vi "NI-USB6509.vi"() -> ()   [LabVIEW 2020]
uses:
  <vilib>/Utility/miscctls.llb/LVPointTypeDef.ctl
  LabVIEW 2020 Toolkits/toolkits_lv2020_32bit/Synchronization.llb/SynchRefs_SetGet.ctl
  LabVIEW 2020 Toolkits/VI Server Toolkit/VI Server Libraries/VI Server_GetControl.llb/VI Server_STR_Get.vi
  LabVIEW 2020 Toolkits/VI Server Toolkit/VI Server Libraries/VI Server_Set Controls.llb/Set STR Control.vi
  LabVIEW 2020 Toolkits/VI Server Toolkit/VI Server Libraries/VI Server_GetControl.llb/VI Server_DAQmx_Device_Get.vi
  LabVIEW 2020 Toolkits/VI Server Toolkit/VI Server Toolkit LV2013.lvlib
panel:
  out "System.Message":string caption="System Message"
  in  "Help":bool
  in  "FP.Hide":bool caption="FrontPanel.Hide"
  in  "EXIT":bool
  in  "Tab.Main":enum32{"Digital I/O", "SETTINGS"}(tab)
  in  "DI.Port.Update":bool
  out "DI.Port.Lines.0:7":u8 caption="Port&Lines 7:0" format="%08b"
  in  "DI.Port":tag="Dev1/port0/line0:7" caption="Port"
  in  "DI.Line":tag="Dev1/port0/line0:7" caption="Line"
  in  "DI.Line.Update":bool caption="Update:"
  in  "DO.Port.Mask.Apply":bool
  in  "DO.Port.Lines.7:0.Mask":u8 caption="Port&Lines 7:0" format="%08b"
  out "DO.Port.State.Verify":bool caption="Verified"
  out "DO.Line.State.Verify":bool caption="Verified"
  in  "DO.Line.State":bool caption="State"
  in  "DO.Line":tag="Dev1/port0/line0:7" caption="Line"
  in  "DO.Port.Update":bool
  in  "DO.Port.Lines.7:0":u8 caption="Port&Lines 7:0" format="%08b"
  in  "DO.Port":tag="Dev1/port0/line0:7" caption="Port"
  in  "DO.Line.Update":bool caption="Update:"
  out "DI.Line.State":bool caption="State"
  in  "VI.WindowsTitle":string caption="Windows Title"
  in  "DAQmx.Device":tag="NI-USB6509" caption="DAQmx: Device"
  in  "UDP.Test.String2.Send":bool
  in  "UDP.Test.String2":string caption="UDP: Test String 2"
  in  "UDP.Port.BC":u16=58433 caption="UDP: Port.BC"
  in  "UDP.Port.RT":u16=58432 caption="UDP: Port.RT"
  in  "UDP.LocalPort.Write":u16=58434 caption="UDP: Local Port.Write"
  in  "UDP.IP.Address":string="234.5.6.7" caption="UDP: IP Address"
  in  "UDP.Test.String1.Send":bool
  in  "UDP.Test.String1":string caption="UDP: Test String 1"
  in  "UDP.Responce.String.Monitor":bool
  out "UDP.ExecEng.Message.String":string caption="UDP: Execution Engine Message String"
  out "error out":errorcluster={"status"=TRUE, "code"=1055, "source"="Property Node in VI Server Toolkit LV2013.lvlib:VI server_Set Control Value from String Format.vi:5200001->DMM6500_UDP_ExecEng_Instruction_APPLY.vi->DMM6500_UDP_MAIN.vi->Keithley2100.vi"}
  in  "error in":errorcluster
  # "Digital Input"
  # "NOTE: Do not use 32 Bit ports configuration!"
  # "Digital Output Port\nMASK"
  # "Instructions:\n1: Active Bit; 0: Masked Bit"
  # "Digital Output"
  # "Multicast IP addresses must be in the 224.0.0.0 to 239.255.255.255 range."
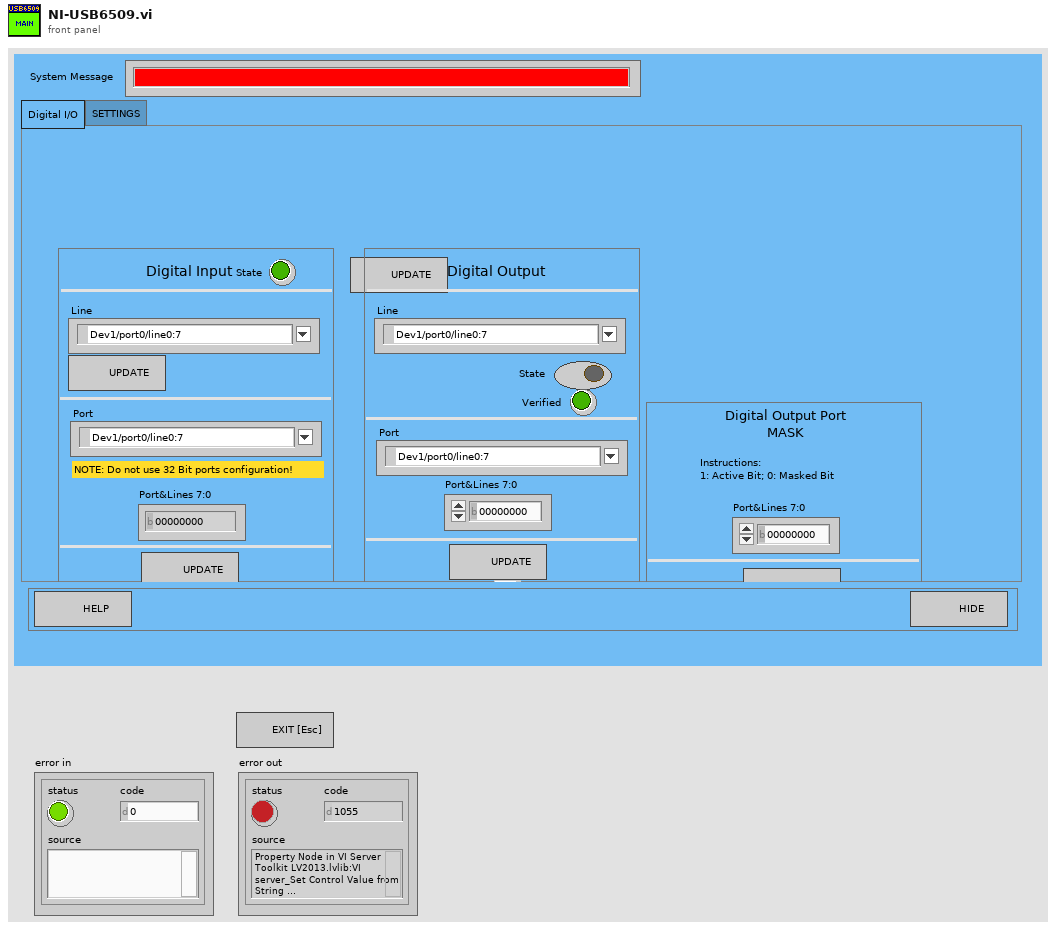
[diagram p1: front panel]
types:
  T1 = typedef "LVPointTypeDef.ctl" = cluster{"Horizontal":i16, "Vertical":i16}
  T2 = typedef "VI Server_RefsCluster.ctl" = cluster{"Labels":string[], "Refs":refnum<vi>[], "VI Ref":refnum<vi>}
  T3 = typedef "SynchRefs_SetGet.ctl" = enum16{"Set", "Get"}
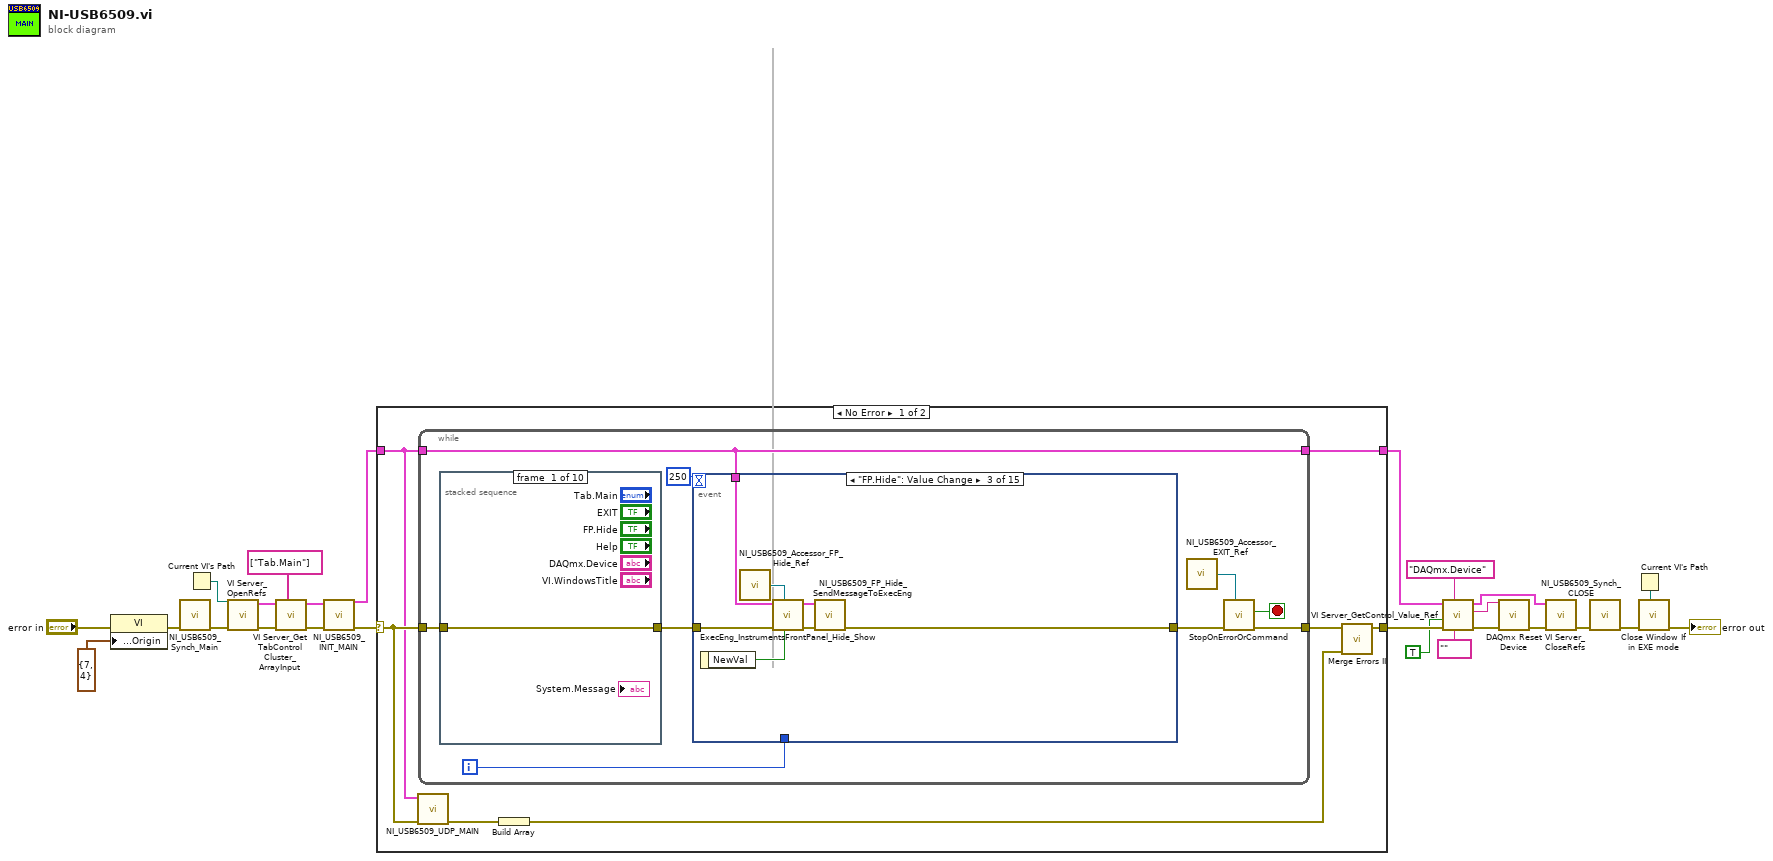
[diagram p0: block diagram]
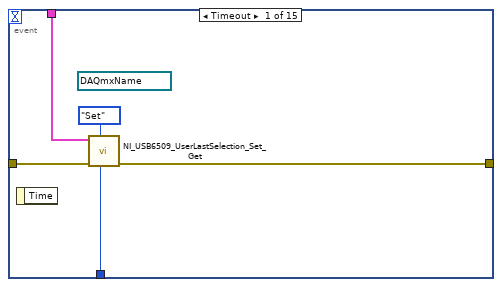
[diagram p2: hidden frame]
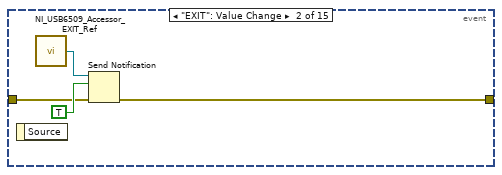
[diagram p3: hidden frame]
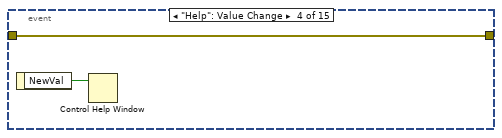
[diagram p4: hidden frame]
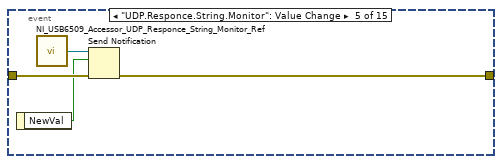
[diagram p5: hidden frame]
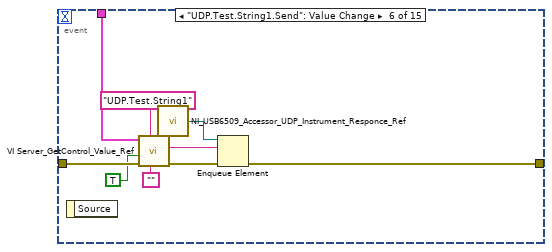
[diagram p6: hidden frame]
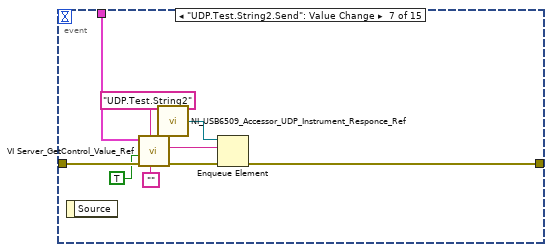
[diagram p7: hidden frame]
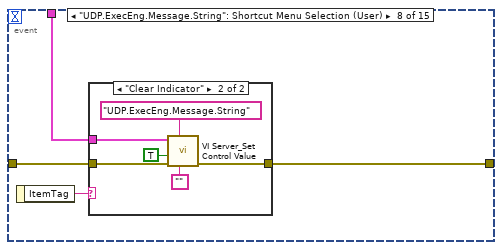
[diagram p8: hidden frame]
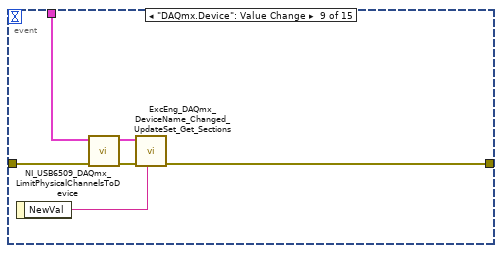
[diagram p10: hidden frame]
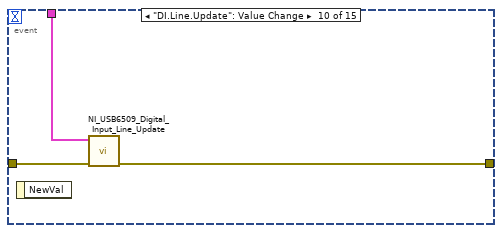
[diagram p11: hidden frame]
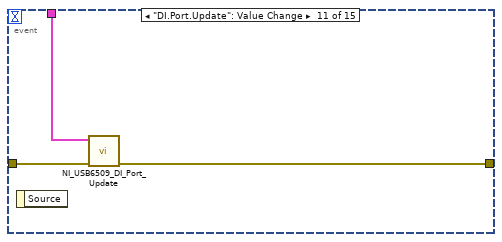
[diagram p12: hidden frame]
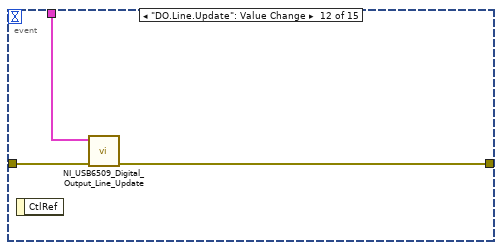
[diagram p13: hidden frame]
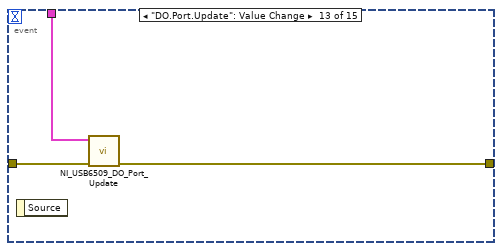
[diagram p14: hidden frame]
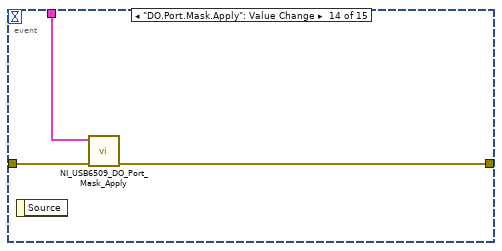
[diagram p15: hidden frame]
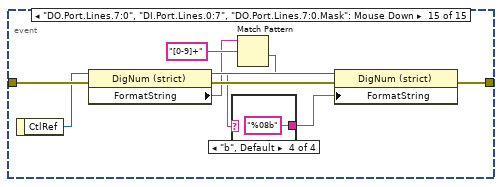
[diagram p16: hidden frame]
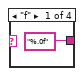
[diagram p17: hidden frame]
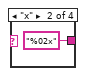
[diagram p18: hidden frame]
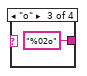
[diagram p19: hidden frame]
diagram:
  n1 = property class="VI"(error in="error in", "Front Panel Window:Origin"=T1 {"Horizontal"=7, "Vertical"=4}) -> (error out=w19:errorcluster)  [unwired: 1 in, 1 out]
  n2 = call "NI_USB6509_Synch_Main.vi"("error in"=w19) -> ("error out"=w20:errorcluster)  [unwired: 10 in]
  n3 = Current VI's Path() -> (path=w24:path)
  n4 = call "VI Server_OpenRefs.vi"("error in"=w20, "VI Path"=w24) -> ("error out"=w21:errorcluster, "VI Server.RefsCluster"=w22:T2)  [unwired: 8 in]
  n5 = call "VI Server_Get TabControl Cluster_ArrayInput.vi"("TabControl Labels[]"=string[] ["Tab.Main"], "error in"=w21, "VI Server Cluster"=w22) -> ("error out"=w18:errorcluster, "VI Server Cluster.OUT"=w17:T2)  [unwired: 7 in]
  n6 = call "NI_USB6509_INIT_MAIN.vi"("error in (no error)"=w18, "VI Server Cluster"=w17) -> ("error out"=w16:errorcluster, "VI Server Cluster DUP"=w15:T2)  [unwired: 8 in]
  n7 = case shown="No Error" w16 {
    selector: w16 -> [w29 w129]
    tunnel: [w30 w129] -> w8
    tunnel: w15 -> [w28 w128]
    tunnel: [w32 w128] -> w5
    frame No Error {
      n8 = call "NI_USB6509_UDP_MAIN.vi"("error in (no error)"=w29, "VI Server.RefsCluster"=w28) -> ("error out"=w27:errorcluster)  [unwired: 9 in]
      n9 = while {
        tunnel: w29 -> [w41]
        tunnel: [w35] -> w31
        tunnel: w28 -> [w37]
        tunnel: [w37] -> w32
        i -> [w38]
        stop <- w34 stop-if-true
        n10 = stacked-sequence {
          tunnel: w41 -> [w127 _ _ _ _ _ _ _ _ _]
          tunnel: [w127 _ _ _ _ _ _ _ _ _] -> w40
          frame #0 {
          }
          frame #1 {
          }
          frame #2 {
          }
          frame #3 {
          }
          frame #4 {
          }
          frame #5 {
          }
          frame #6 {
          }
          frame #7 {
          }
          frame #8 {
          }
          frame #9 {
          }
        }
        n11 = event shown="[2] \"FP.Hide\": Value Change" {
          selector: _ -> [_ _ _ _ _ _ _ _ _ _ _ _ _ _ _]
          dyn-events: _ -> [_ _ _ _ _ _ _ _ _ _ _ _ _ _ _]
          timeout: 250 -> [_ _ _ _ _ _ _ _ _ _ _ _ _ _ _]
          tunnel: w40 -> [w45 w47 w56 w59 w63 w72 w81 w85 w98 w101 w104 w107 w110 w113 w122]
          tunnel: w38 -> [w44 _ _ _ _ _ _ _ _ _ _ _ _ _ _]
          tunnel: [w42 w49 w57 w59 w61 w70 w79 w83 w95 w100 w102 w105 w108 w111 w119] -> w36
          tunnel: w37 -> [w43 _ w53 _ _ w69 w78 w82 w97 w99 w103 w106 w109 w112 _]
          event Timeout {
            (unwired) refnum<vi> refnum ("DAQmx.Device")
            n12 = event-data() -> ()  [unwired: 1 in, 1 out]
            n13 = call "NI_USB6509_UserLastSelection_Set_Get.vi"("LoopCounter"=w44, "SynchRefs.Set/Get"=SynchRefs_SetGet."Set", "error in"=w45, "VI Server.RefsCluster"=w43) -> ("error out"=w42:errorcluster)  [unwired: 6 in, 1 out]
          }
          event "EXIT": Value Change {
            n14 = event-data() -> ()  [unwired: 1 in, 1 out]
            n15 = call "NI_USB6509_Accessor_EXIT_Ref.vi"() -> ("EXIT"=w50:refnum<notifier>)  [unwired: 6 in]
            n16 = Send Notification(notification=TRUE, notifier=w50, error in (no error)=w47) -> (error out=w49:errorcluster)  [unwired: 1 out]
          }
          event "FP.Hide": Value Change {
            n17 = event-data() -> ("NewVal"=w51:bool)  [unwired: 1 in]
            n18 = call "NI_USB6509_Accessor_FP_Hide_Ref.vi"() -> ("FP.Hide"=w52:refnum<notifier>)  [unwired: 6 in]
            n19 = call "ExecEng_InstrumentsFrontPanel_Hide_Show.vi"("FP.Hide/Show"=w51, "FP.State"=w52, "error in (no error)"=w56, "VI Server Cluster"=w53) -> ("error out"=w55:errorcluster, "VI Server Cluster DUP"=w54:T2)  [unwired: 6 in]
            n20 = call "NI_USB6509_FP_Hide_SendMessageToExecEng.vi"("error in (no error)"=w55, "VI Server Cluster"=w54) -> ("error out"=w57:errorcluster)  [unwired: 9 in]
          }
          event "Help": Value Change {
            n21 = event-data() -> ("NewVal"=w58:bool)  [unwired: 1 in]
            n22 = Control Help Window(1:w58) -> ()  [unwired: 1 in]
          }
          event "UDP.Responce.String.Monitor": Value Change {
            n23 = event-data() -> ("NewVal"=w60:bool)  [unwired: 1 in]
            n24 = call "NI_USB6509_Accessor_UDP_Responce_String_Monitor_Ref.vi"() -> ("UDP.ExecEng.Command.String.Monitor"=w62:refnum<notifier>)  [unwired: 6 in]
            n25 = Send Notification(notification=w60, notifier=w62, error in (no error)=w63) -> (error out=w61:errorcluster)  [unwired: 1 out]
          }
          event "UDP.Test.String1.Send": Value Change {
            n26 = event-data() -> ()  [unwired: 1 in, 1 out]
            n27 = call-poly "VI Server_GetControl_Value_Ref.vi"("DataType"="", "Control.Label"="UDP.Test.String1", "error in"=w72, "SingleInstance"=TRUE, "VI Server.RefsCluster"=w69) -> ("error out"=w71:errorcluster, "Value"=w64:string)  [unwired: 3 in, 2 out]
            n28 = call "NI_USB6509_Accessor_UDP_Instrument_Responce_Ref.vi"() -> ("UDP.Instrument.Responce.Q"=w65:refnum<queue>)  [unwired: 6 in]
            n29 = Enqueue Element(queue=w65, element=w64, error in (no error)=w71) -> (error out=w70:errorcluster)  [unwired: 1 in, 2 out]
          }
          event "UDP.Test.String2.Send": Value Change {
            n30 = event-data() -> ()  [unwired: 1 in, 1 out]
            n31 = call-poly "VI Server_GetControl_Value_Ref.vi"("DataType"="", "Control.Label"="UDP.Test.String2", "error in"=w81, "SingleInstance"=TRUE, "VI Server.RefsCluster"=w78) -> ("error out"=w80:errorcluster, "Value"=w73:string)  [unwired: 3 in, 2 out]
            n32 = call "NI_USB6509_Accessor_UDP_Instrument_Responce_Ref.vi"() -> ("UDP.Instrument.Responce.Q"=w74:refnum<queue>)  [unwired: 6 in]
            n33 = Enqueue Element(queue=w74, element=w73, error in (no error)=w80) -> (error out=w79:errorcluster)  [unwired: 1 in, 2 out]
          }
          event "UDP.ExecEng.Message.String": Shortcut Menu Selection (User) {
            n34 = event-data() -> ("ItemTag"=w84:string)  [unwired: 1 in]
            n35 = case shown="\"Clear Indicator\"" w84 {
              tunnel: w85 -> [w86 w92]
              tunnel: [w86 w91] -> w83
              tunnel: w82 -> [_ w90]
              frame "", Default {
              }
              frame "Clear Indicator" {
                n36 = call-poly "VI Server_Set Control Value.vi"("New Value"="", "Label"="UDP.ExecEng.Message.String" ("Control.Label"), "error in"=w92, "Single Instance (T)"=TRUE ("SingleInstance"), "VI Server Cluster"=w90) -> ("error out"=w91:errorcluster)  [unwired: 4 in, 2 out]
              }
            }
          }
          event "DAQmx.Device": Value Change {
            n37 = event-data() -> ("NewVal"=w93:tag)  [unwired: 1 in]
            n38 = call "NI_USB6509_DAQmx_LimitPhysicalChannelsToDevice.vi"("error in (no error)"=w98, "VI Server Cluster"=w97) -> ("error out"=w96:errorcluster, "VI Server Cluster.DUP"=w94:T2)  [unwired: 7 in, 1 out]
            n39 = call "ExcEng_DAQmx_DeviceName_Changed_UpdateSet_Get_Sections.vi"("DAQmx.Device"=w93, "error in (no error)"=w96, "VI Server Cluster"=w94) -> ("error out"=w95:errorcluster)  [unwired: 8 in]
          }
          event "DI.Line.Update": Value Change {
            n40 = event-data() -> ()  [unwired: 1 in, 1 out]
            n41 = call "NI_USB6509_Digital_Input_Line_Update.vi"("error in (no error)"=w101, "VI Server Cluster"=w99) -> ("error out"=w100:errorcluster)  [unwired: 9 in]
          }
          event "DI.Port.Update": Value Change {
            n42 = event-data() -> ()  [unwired: 1 in, 1 out]
            n43 = call "NI_USB6509_DI_Port_Update.vi"("error in (no error)"=w104, "VI Server Cluster"=w103) -> ("error out"=w102:errorcluster)  [unwired: 9 in]
          }
          event "DO.Line.Update": Value Change {
            n44 = event-data() -> ()  [unwired: 1 in, 1 out]
            n45 = call "NI_USB6509_Digital_Output_Line_Update.vi"("error in (no error)"=w107, "VI Server Cluster"=w106) -> ("error out"=w105:errorcluster)  [unwired: 9 in]
          }
          event "DO.Port.Update": Value Change {
            n46 = event-data() -> ()  [unwired: 1 in, 1 out]
            n47 = call "NI_USB6509_DO_Port_Update.vi"("error in (no error)"=w110, "VI Server Cluster"=w109) -> ("error out"=w108:errorcluster)  [unwired: 9 in]
          }
          event "DO.Port.Mask.Apply": Value Change {
            n48 = event-data() -> ()  [unwired: 1 in, 1 out]
            n49 = call "NI_USB6509_DO_Port_Mask_Apply.vi"("error in (no error)"=w113, "VI Server Cluster"=w112) -> ("error out"=w111:errorcluster)  [unwired: 9 in]
          }
          event "DO.Port.Lines.7:0", "DI.Port.Lines.0:7", "DO.Port.Lines.7:0.Mask": Mouse Down {
            n50 = event-data() -> ("CtlRef"=w121:refnum<vi>)  [unwired: 1 in]
            n51 = property class="DigNum (strict)"(reference=w121, error in=w122) -> (reference out=w118:refnum<vi>, error out=w120:errorcluster, "FormatString"=w115:string)
            n52 = Match Pattern(string=w115, regular expression="[0-9]+") -> (after substring=w114:string)  [unwired: 1 in, 3 out]
            n53 = case shown="\"b\", Default" w114 {
              tunnel: ["%.0f" "%02x" "%02o" "%08b"] -> w117
              frame "f" {
              }
              frame "x" {
              }
              frame "o" {
              }
              frame "b", Default {
              }
            }
            n54 = property class="DigNum (strict)"(reference=w118, error in=w120, "FormatString"=w117) -> (error out=w119:errorcluster)  [unwired: 1 out]
          }
        }
        n55 = call "NI_USB6509_Accessor_EXIT_Ref.vi"() -> ("EXIT"=w33:refnum<notifier>)  [unwired: 6 in]
        n56 = call "StopOnErrorOrCommand.vi"("STOP"=w33, "error in (no error)"=w36) -> ("error out"=w35:errorcluster, "STOP"=w34:bool)  [unwired: 8 in]
      }
      n57 = Build Array(w27) -> (w26:errorcluster[])
      n58 = call "Merge Errors II.vi"("error array in"=w26, "error in 1 (no error)"=w31) -> ("error out.DUP"=w30:errorcluster)  [unwired: 4 in, 1 out]
    }
    frame Error {
    }
  }
  n59 = call-poly "VI Server_GetControl_Value_Ref.vi"("DataType"=tag "" ("DAQmx.Device"), "Control.Label"="DAQmx.Device", "error in"=w8, "SingleInstance"=TRUE, "VI Server.RefsCluster"=w5) -> ("error out"=w11:errorcluster, "Value"=w12:tag, "VI Server.RefsCluster.DUP"=w6:T2)  [unwired: 3 in, 1 out]
  n60 = call <vilib>:"DAQmx Reset Device.vi"("device in"=w12, "error in"=w11) -> ("error out"=w7:errorcluster)  [unwired: 13 in]
  n61 = call "VI Server_CloseRefs.vi"("error in"=w7, "VI Server.RefsCluster"=w6) -> ("error out"=w14:errorcluster)  [unwired: 9 in]
  n62 = call "NI_USB6509_Synch_CLOSE.vi"("error in"=w14) -> ("error out"=w3:errorcluster)  [unwired: 10 in]
  n63 = Current VI's Path() -> (path=w1:path)
  n64 = call "Close Window If in EXE mode.vi"("TopLevelVI Path"=w1, "error in"=w3) -> ("error out"=→"error out":errorcluster)  [unwired: 9 in]
